vi "CRYRemove Report G-View Info.vi"(11 "DataView_Info Array":T1[](array[typedef])) -> (0 "DataView_Info Array Except Report out":T1[](array[typedef]), 3 "DataView_Info Array out":T1[](array[typedef]))   [LabVIEW 2013]
uses:
  Control/Graph Main Info Cluster.ctl
  Control/SplitterBar.ctl
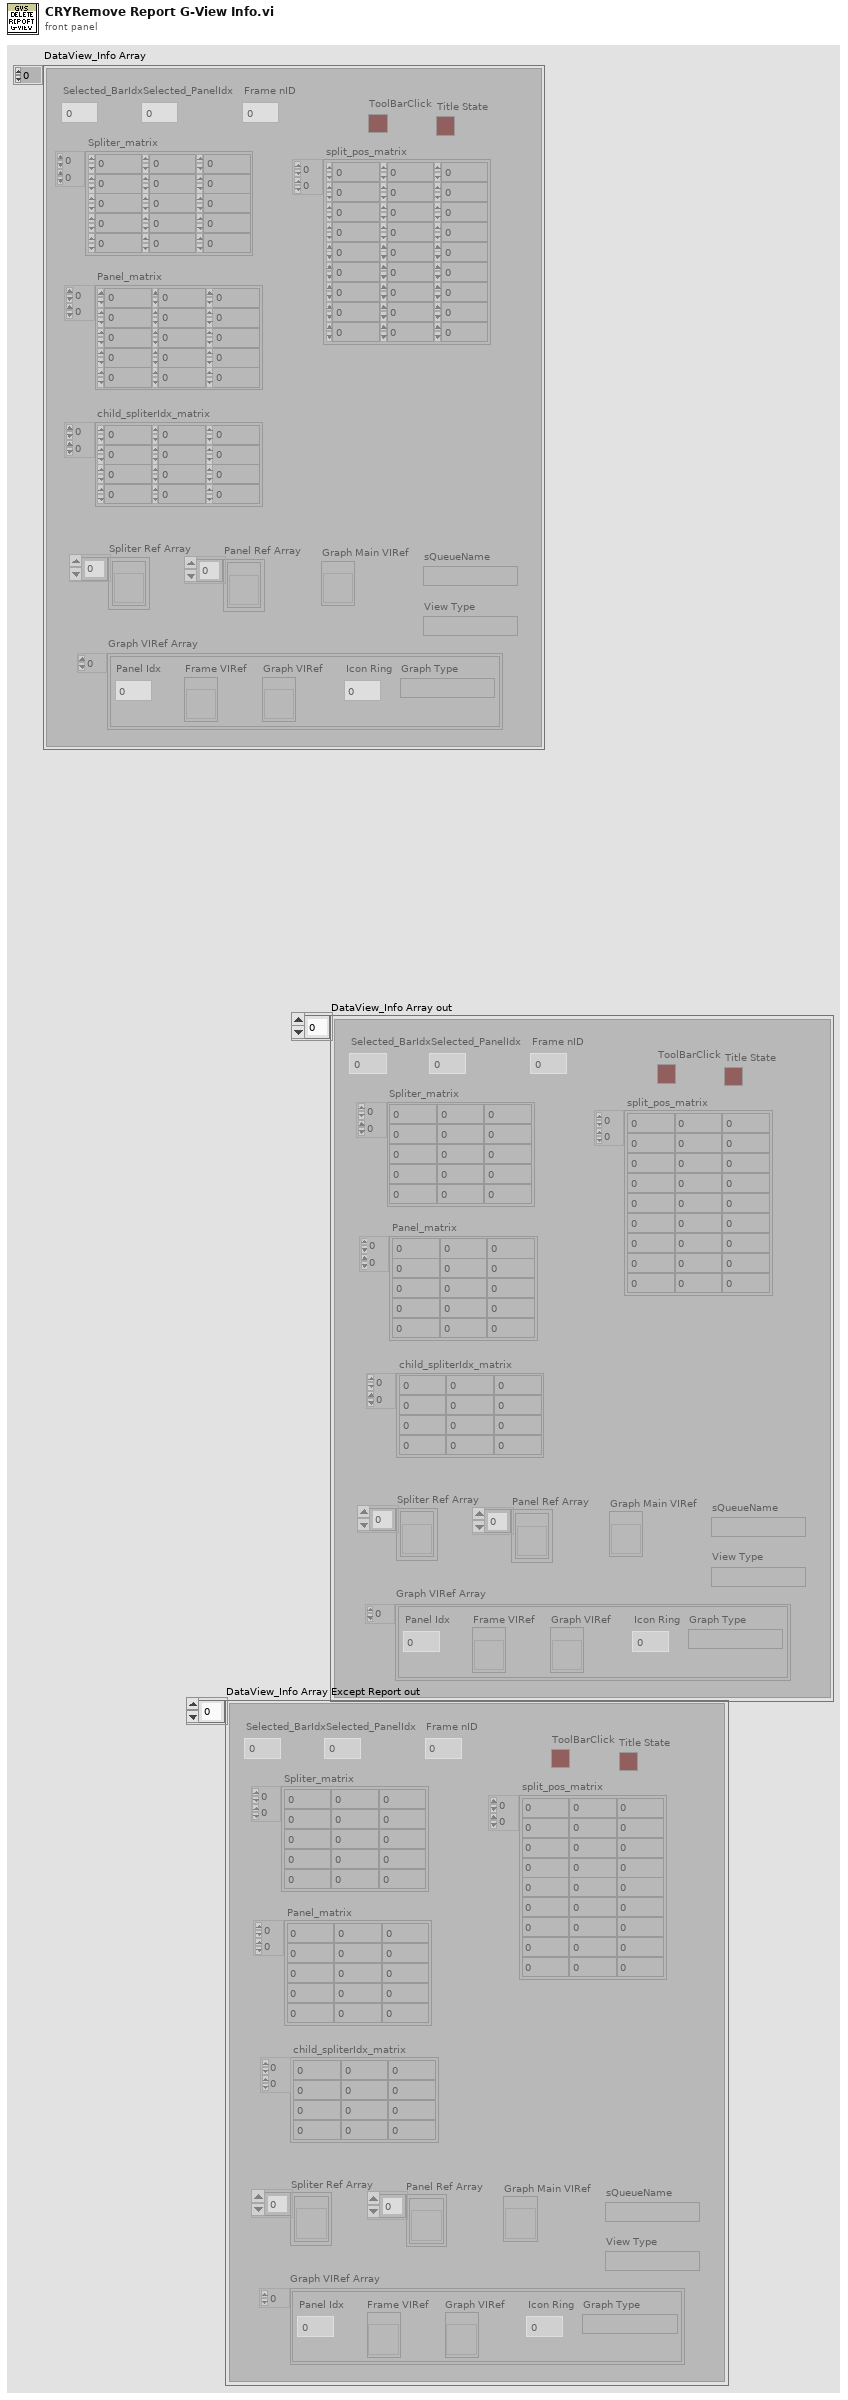
[diagram p1: front panel]
types:
  T1 = typedef "Graph Main Info Cluster.ctl" = cluster{"Selected_BarIdx":i32, "Selected_PanelIdx":i32, "Graph Main VIRef":refnum<vi>, "ToolBarClick":bool, "Spliter Ref Array":refnum<vi>[], "Panel Ref Array":refnum<vi>[], "Spliter_matrix":i32[][], "Panel_matrix":i32[][], "child_spliterIdx_matrix":i32[][], "split_pos_matrix":i32[][], "Title State":bool, "sQueueName":string, "Frame nID":i32, "Graph VIRef Array":cluster{"Graph VIRef":refnum<vi>, "Panel Idx":i32, "Frame VIRef":refnum<vi>, "Icon Ring":i32, "Graph Type":string}[], "View Type":string}
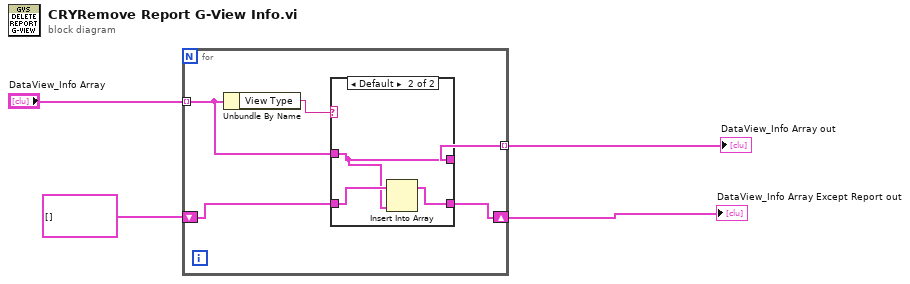
[diagram p0: block diagram]
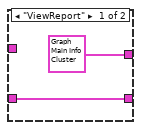
[diagram p2: hidden frame]
diagram:
  n1 = for {
    tunnel: "DataView_Info Array" -> [w8] mode=indexing
    tunnel: [w7] -> w3 mode=indexing
    shift-right: [w5] -> w1
    shift-left: T1[] [] ("DataView_Info Array") -> [w6]
    n2 = Unbundle By Name(w8) -> ("View Type"=w9:string)
    n3 = case shown="Default" w9 {
      tunnel: w8 -> [_ w13]
      tunnel: [T1 {"Selected_BarIdx"=0, "Selected_PanelIdx"=0, "Graph Main VIRef"=refnum, "ToolBarClick"=FALSE, "Spliter Ref Array"=[], "Panel Ref Array"=[], "Spliter_matrix"=[], "Panel_matrix"=[], "child_spliterIdx_matrix"=[], "split_pos_matrix"=[], "Title State"=FALSE, "sQueueName"="", "Frame nID"=0, "Graph VIRef Array"=[], "View Type"=""} ("Cluster") w13] -> w7
      tunnel: w6 -> [w10 w14]
      tunnel: [w10 w12] -> w5
      frame "ViewReport" {
      }
      frame Default {
        n4 = Insert Into Array(array=w14, new element=w13) -> (w12:T1[])  [unwired: 1 in]
      }
    }
  }
  "DataView_Info Array out" <- w3
  "DataView_Info Array Except Report out" <- w1
